vi "Create DVRs.vi"(8 "error in (no error)":errorcluster, 11 "Engine in":refnum<class "Engine.lvclass">) -> (0 "error out":errorcluster, 3 "Engine out":refnum<class "Engine.lvclass">)   [LabVIEW 2023, in "Engine.lvlib" / "Engine.lvclass"]
uses:
  Library/Engine.lvclass
  Library/Engine.lvclass/Engine.ctl
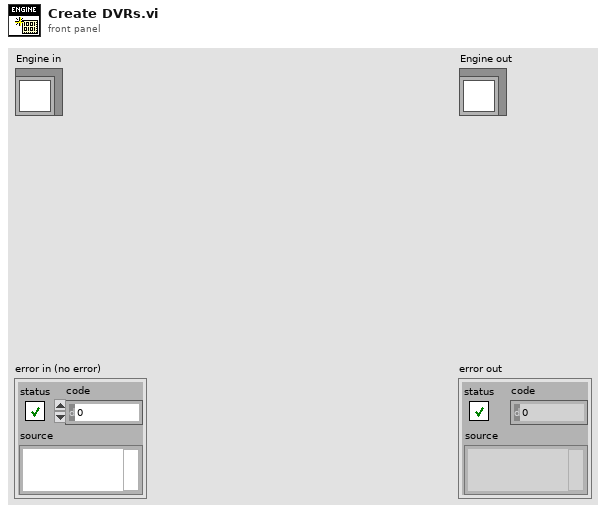
[diagram p1: front panel]
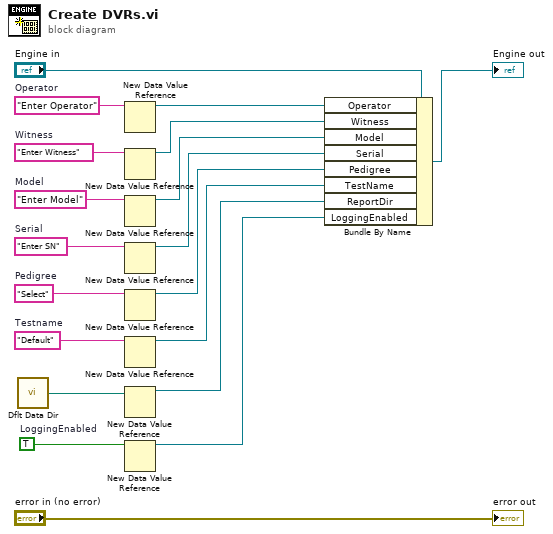
[diagram p0: block diagram]
diagram:
  w1 = TRUE  # LoggingEnabled
  w11 = "Default"  # Testname
  w10 = "Select"  # Pedigree
  w12 = "Enter SN"  # Serial
  w13 = "Enter Model"  # Model
  w14 = "Enter Witness"  # Witness
  w17 = "Enter Operator"  # Operator
  n1 = call <vilib>:"Dflt Data Dir.vi"() -> ("App:Default Data Directory"=w4:path)
  n2 = New Data Value Reference(data value=w17) -> (data value reference=w15:refnum<data-value>)  [unwired: 1 in, 1 out]
  n3 = New Data Value Reference(data value=w14) -> (data value reference=w9:refnum<data-value>)  [unwired: 1 in, 1 out]
  n4 = New Data Value Reference(data value=w13) -> (data value reference=w8:refnum<data-value>)  [unwired: 1 in, 1 out]
  n5 = New Data Value Reference(data value=w12) -> (data value reference=w7:refnum<data-value>)  [unwired: 1 in, 1 out]
  n6 = New Data Value Reference(data value=w10) -> (data value reference=w6:refnum<data-value>)  [unwired: 1 in, 1 out]
  n7 = New Data Value Reference(data value=w11) -> (data value reference=w5:refnum<data-value>)  [unwired: 1 in, 1 out]
  n8 = New Data Value Reference(data value=w4) -> (data value reference=w3:refnum<data-value>)  [unwired: 1 in, 1 out]
  n9 = New Data Value Reference(data value=w1) -> (data value reference=w2:refnum<data-value>)  [unwired: 1 in, 1 out]
  n10 = Bundle By Name(cluster="Engine in", "Operator"=w15, "Witness"=w9, "Model"=w8, "Serial"=w7, "Pedigree"=w6, "TestName"=w5, "ReportDir"=w3, "LoggingEnabled"=w2) -> (→"Engine out":refnum<class "Engine.lvclass">)
  "error out" <- "error in (no error)"
